vi "FringeTrackerOpenSynchronization.vi"(9 "error in (no error)":errorcluster) -> (2 "FringeTrackerSynchro":T1, 6 "error out":errorcluster)   [LabVIEW 2009]
uses:
  Controls/FringeTrackerSynchro.ctl
  Controls/FringTrackerCommand.ctl
  Controls/FringeTrackerData.ctl
  Nicmos/Controls/NICMOS.READOUT.ctl
  Controls/FringeTrackerState.ctl
  Controls/FringeTrackerInfo.ctl
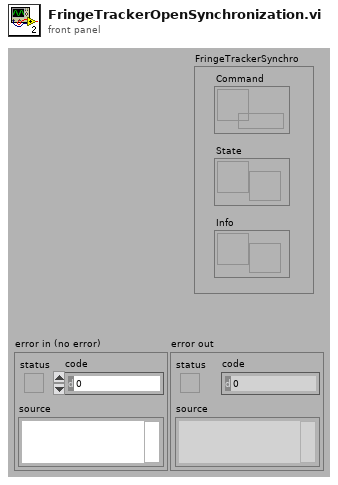
[diagram p1: front panel]
types:
  T1 = typedef "FringeTrackerSynchro.ctl" = cluster{"Command":refnum<queue>, "State":refnum<notifier>, "Info":refnum<notifier>}
  T2 = typedef "FringeTrackerInfo.ctl" = cluster{"Readout":T3, "OPD stroke":dbl[unit], "OPD per pixel":dbl[unit]}
  T3 = typedef "NICMOS.READOUT.ctl" = cluster{"Readout":i32, "Deglitch":i32, "Framerate":dbl[unit], "Bank":i32}
  T4 = typedef "FringeTrackerState.ctl" = enum16{"IDLING", "CONFIGURING", "SCANNING", "STOPPING"}
  T5 = typedef "FringTrackerCommand.ctl" = cluster{"Command":enum16{"IDLE", "SCAN", "QUIT"}, "FringeScannerData":T6}
  T6 = typedef "FringeTrackerData.ctl" = cluster{"Readout":T3, "Wavelength":dbl[unit], "Frame per fringe":dbl, "Autcollimation":bool}
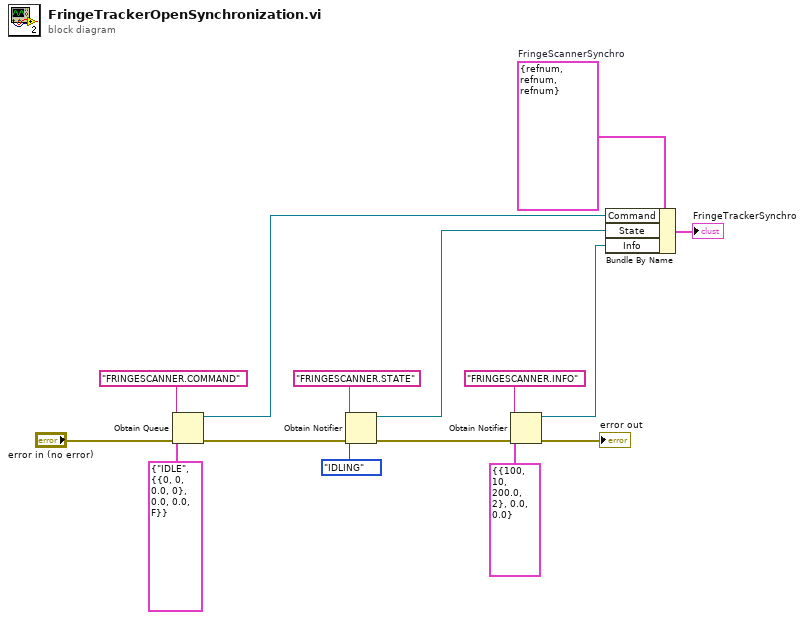
[diagram p0: block diagram]
diagram:
  w9 = T1 {"Command"=refnum, "State"=refnum, "Info"=refnum}  # FringeScannerSynchro
  n1 = Obtain Queue(name (unnamed)="FRINGESCANNER.COMMAND", element data type=T5 {"Command"=enum."IDLE", "FringeScannerData"={"Readout"={"Readout"=0, "Deglitch"=0, "Framerate"=0.0, "Bank"=0}, "Wavelength"=0.0, "Frame per fringe"=0.0, "Autcollimation"=FALSE}} ("FringeScannerCommand"), error in (no error)="error in (no error)") -> (queue out=w8:refnum<queue>, error out=w12:errorcluster)  [unwired: 2 in, 1 out]
  n2 = Obtain Notifier(name (unnamed)="FRINGESCANNER.STATE", notification data type=FringeTrackerState."IDLING" ("FringeScannerState"), error in (no error)=w12) -> (notifier out=w7:refnum<notifier>, error out=→"error out":errorcluster)  [unwired: 1 in, 1 out]
  n3 = Obtain Notifier(name (unnamed)="FRINGESCANNER.INFO", notification data type=T2 {"Readout"={"Readout"=100, "Deglitch"=10, "Framerate"=200.0, "Bank"=2}, "OPD stroke"=0.0, "OPD per pixel"=0.0} ("FringeScannerInfo")) -> (notifier out=w1:refnum<notifier>)  [unwired: 2 in, 2 out]
  n4 = Bundle By Name(cluster=w9, "Command"=w8, "State"=w7, "Info"=w1) -> (→"FringeTrackerSynchro":T1)
